vi "Esercizio lezione 8-4 Lavoro Client.vi"(2 "Server Address":string="localhost", 3 "Port":u16=6340 min=1025 step=1) -> (0 "Numero":i32, 1 "read string":string)   [LabVIEW 2012]
doc: "© Copyright M. Ferrari 2010"
panel:
  # "CLIENT: legge una stringa inviata dal Server"
  # "Realizzare un server che al posto di una stringa permetta di inviare un valore numerico\nintero (I32) ad un client. La parte relativa al client dovrà visualizzare sia il valore numerico \nche la stringa letta ( byte stream). Interpretare i risultati provando ad inviare alcuni valori\nnumerici, ad esempio 3; 15; 255; -1."
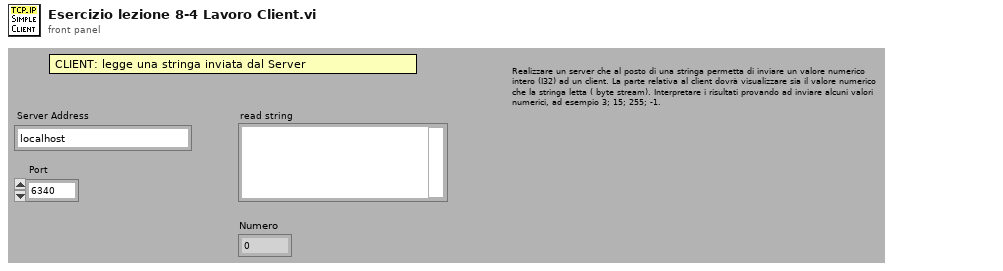
[diagram p1: front panel]
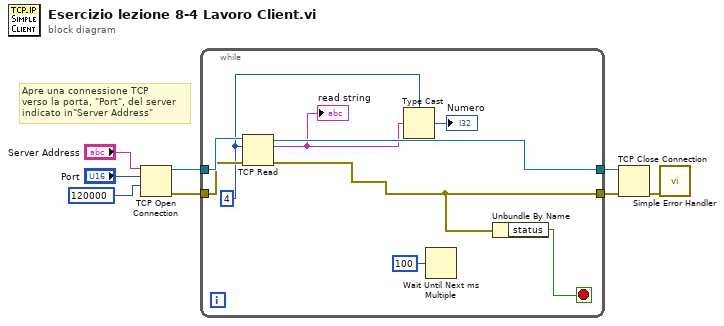
[diagram p0: block diagram]
diagram:
  # "Apre una connessione TCP\nverso la porta, \"Port\", del server\nindicato in\"Server Address\""
  n1 = TCP Open Connection(address="Server Address", remote port or service name="Port", timeout ms (60000)=120000) -> (connection ID=w5:refnum<k5>, error out=w6:errorcluster)  [unwired: 2 in]
  n2 = while {
    tunnel: w5 -> [w15]
    tunnel: w6 -> [w14]
    tunnel: [w11] -> w2
    tunnel: [w12] -> w1
    stop <- w16 stop-if-true
    w13 = 4 ("bytes to read")
    n3 = TCP Read(connection ID=w15, bytes to read=w13, error in (no error)=w14) -> (connection ID out=w11:refnum<k5>, data out=w10:string, error out=w12:errorcluster)  [unwired: 2 in]
    "read string" <- w10
    n4 = Type Cast(type=w13, x=w10) -> (*(type *) &x=→"Numero":i32)
    n5 = Wait Until Next ms Multiple(millisecond multiple=u32 100) -> ()  [unwired: 1 out]
    n6 = Unbundle By Name(w12) -> ("status"=w16:bool)
  }
  n7 = TCP Close Connection(connection ID=w2, error in (no error)=w1) -> (error out=w4:errorcluster)  [unwired: 1 in, 1 out]
  n8 = call <vilib>:"Simple Error Handler.vi"("error in (no error)"=w4) -> ()  [unwired: 4 in, 5 out]
